vi "Handle GET.vi"(8 "error in (no error)":errorcluster, 9 "data":variant, 10 "parameter":string, 11 "Instrument in":refnum<class "Instrument.lvclass">) -> (0 "error out":errorcluster, 2 "data out":variant, 3 "Instrument out":refnum<class "Instrument.lvclass">)   [LabVIEW 2019, in "Instrument.lvlib" / "Instrument.lvclass"]
uses:
  Instrument.lvclass
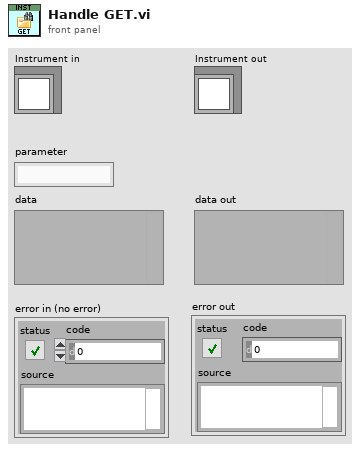
[diagram p1: front panel]
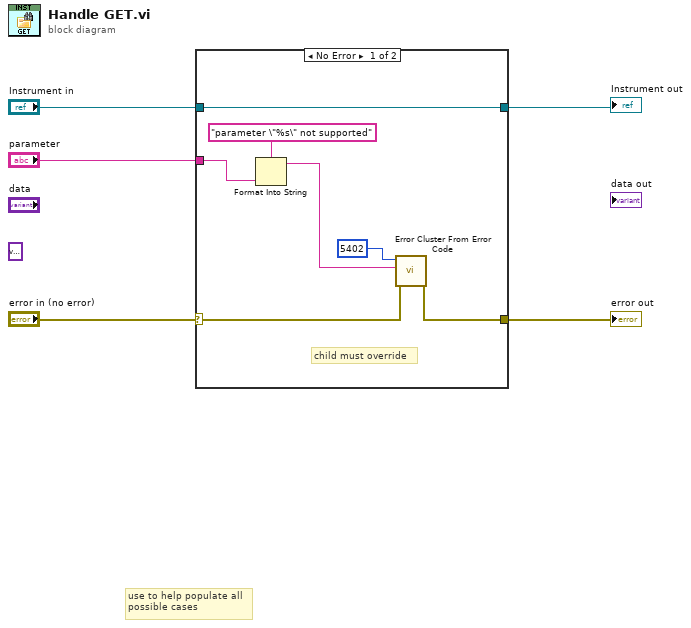
[diagram p0: block diagram]
diagram:
  (unwired) variant ("data")
  # "use to help populate all\npossible cases"
  n1 = case shown="No Error" "error in (no error)" {
    selector: "error in (no error)" -> [w10 w13]
    tunnel: [w12 w14] -> w5
    tunnel: "Instrument in" -> [w12 w14]
    tunnel: [w9 w13] -> w3
    tunnel: "parameter" -> [w8 _]
    frame No Error {
      # "child must override"
      n2 = Format Into String(format string="parameter \"%s\" not supported" ("error message (\"\")"), w8) -> (resulting string=w6:string)  [unwired: 2 in, 1 out]
      n3 = call <vilib>:"Error Cluster From Error Code.vi"("error in (no error)"=w10, "error message (\"\")"=w6, "error code (0)"=5402) -> ("error out"=w9:errorcluster)  [unwired: 6 in]
    }
    frame Error {
    }
  }
  "Instrument out" <- w5
  "error out" <- w3
